vi "18.2.2 Matching-Identification.vi"() -> ()   [LabVIEW 2017]
doc: "This example illustrates the use of the horizontal clamp tool. You can draw a region of inspection that contains at least two edges in the image. The VI measures the distance between the first and last edges."
uses:
  <vilib>/vision/NI_Vision_Development_Module.lvlib
panel:
  out "Score":i32[](array[numeric])
  out "Match":bool[](array[boolean])
  out "TMP":T1(plugin-control)
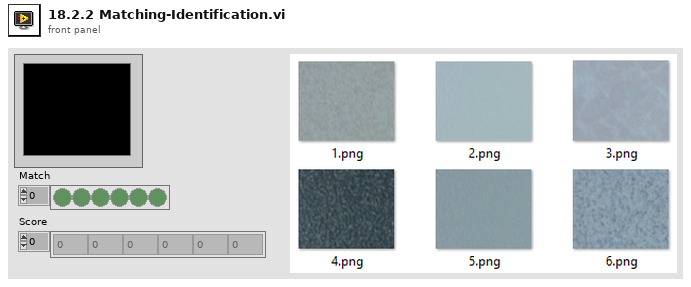
[diagram p1: front panel]
types:
  T1 = typedef "IMAQ Image.ctl" = refnum<image>
  T2 = typedef "Image Type" = u32
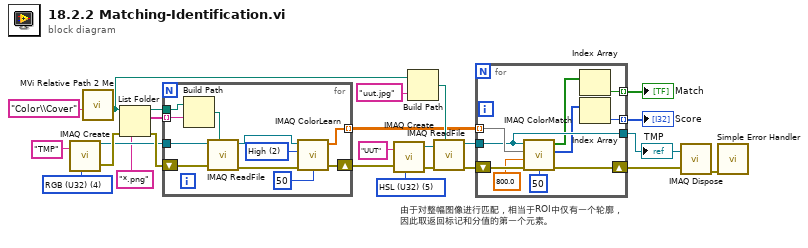
[diagram p0: block diagram]
diagram:
  w16 = T2 5 items=["Grayscale (U8)", "Grayscale (I16)", "Grayscale (SGL)", "Complex (CSG)", "RGB (U32)", "HSL (U32)", "RGB (U64)", "Grayscale (U16)"] ("Image Type")
  w22 = T2 4 items=["Grayscale (U8)", "Grayscale (I16)", "Grayscale (SGL)", "Complex (CSG)", "RGB (U32)", "HSL (U32)", "RGB (U64)", "Grayscale (U16)"] ("Image Type")
  # "由于对整幅图像进行匹配，相当于ROI中仅有一个轮廓，\n因此取返回标记和分值的第一个元素。"
  n1 = call "IMAQ Create"("Image Name"="TMP", "Image Type"=w22) -> ("New Image"=w17:T1, "error out"=w19:errorcluster)  [unwired: 3 in]
  n2 = call "MVi Relative Path 2 Me.vi"("Relative Path"="Color\\Cover" ("name or relative path")) -> ("Appended Dir"=w13:path)  [unwired: 5 in, 1 out]
  n3 = List Folder(path=w13, pattern="*.png", error in=w19) -> (path out=w20:path, filenames=w21:string[], error out=w18:errorcluster)  [unwired: 1 in, 1 out]
  n4 = for {
    tunnel: w21 -> [w29] mode=indexing
    tunnel: w20 -> [w28]
    shift-right: [w31] -> w8
    shift-left: w18 -> [w33]
    tunnel: w17 -> [w32]
    tunnel: [w30] -> w6 mode=indexing
    w34 = u32 2 items=["Low", "Medium", "High"] ("Color Sensitivity")
    n5 = Build Path(base path=w28, name or relative path=w29) -> (appended path=w27:path)
    n6 = call "IMAQ ReadFile"("File Path"=w27, "error in (no error)"=w33, "Image"=w32) -> ("error out"=w35:errorcluster, "Image Out"=w36:T1)  [unwired: 4 in, 3 out]
    n7 = call "IMAQ ColorLearn"("Image"=w36, "Color Sensitivity"=w34, "Learn Saturation Threshold"=50, "error in (no error)"=w35) -> ("Color Spectrum"=w30:dbl[], "error out"=w31:errorcluster)  [unwired: 4 in]
  }
  n8 = call "IMAQ Create"("Image Name"="UUT", "Image Type"=w16, "error in (no error)"=w8) -> ("New Image"=w11:T1, "error out"=w10:errorcluster)  [unwired: 2 in]
  n9 = Build Path(base path=w13, name or relative path="uut.jpg") -> (appended path=w9:path)
  n10 = call "IMAQ ReadFile"("File Path"=w9, "error in (no error)"=w10, "Image"=w11) -> ("error out"=w7:errorcluster, "Image Out"=w5:T1)  [unwired: 4 in, 3 out]
  n11 = for {
    shift-right: [w44] -> w4
    shift-left: w7 -> [w46]
    tunnel: w6 -> [w45] mode=indexing
    tunnel: w5 -> [w43]
    tunnel: [w41] -> w2 mode=indexing
    tunnel: [w43] -> w3
    tunnel: [w39] -> w1 mode=indexing
    n12 = call "IMAQ ColorMatch"("Image"=w43, "Color Spectrum"=w45, "Match Saturation Threshold"=50, "Minimum Match Score"=800.0, "error in (no error)"=w46) -> ("Match Flag"=w42:bool[], "Match Score"=w40:i32[], "error out"=w44:errorcluster)  [unwired: 1 in, 1 out]
    n13 = Index Array(array=w42) -> (element=w41:bool)  [unwired: 1 in]
    n14 = Index Array(array=w40) -> (element=w39:i32)  [unwired: 1 in]
  }
  "TMP" <- w3
  "Match" <- w2
  "Score" <- w1
  n15 = call "IMAQ Dispose"("Image"=w3, "error in (no error)"=w4) -> ("error out"=w25:errorcluster)  [unwired: 4 in]
  n16 = call <vilib>:"Simple Error Handler.vi"("error in (no error)"=w25) -> ()  [unwired: 4 in, 5 out]
